vi "Get Data per Frequency at Pin Point Index.vi"(10 "Pin Point Index":i32, 11 "Full Data per Freq":string[][](array[string])) -> (3 "Focused Data":string[][](array[string]))   [LabVIEW 2023, in "FPT_Compression UI.lvlib"]
uses:
  FPT_Compression UI.lvlib
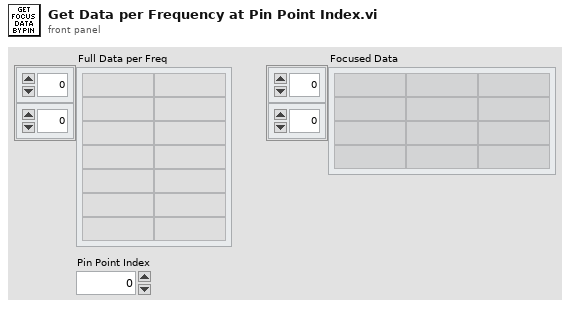
[diagram p1: front panel]
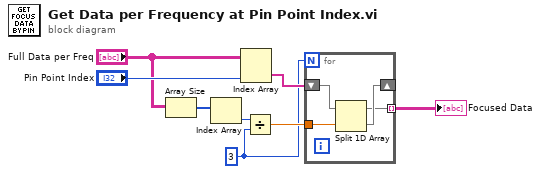
[diagram p0: block diagram]
diagram:
  w2 = 3 ("y")
  n1 = Array Size(array="Full Data per Freq") -> (size(s)=w3:i32[])
  n2 = Index Array(array=w3) -> (element=w6:i32)  [unwired: 1 in]
  n3 = Index Array(array="Full Data per Freq", index (col)="Pin Point Index") -> (element=w7:string[])  [unwired: 1 in]
  n4 = Divide(x=w6, y=w2) -> (x/y=w8:dbl)
  n5 = for {
    N: w2 -> [_]
    tunnel: [w11] -> w1 mode=indexing
    tunnel: w8 -> [w10]
    shift-right: [w12] -> _
    shift-left: w7 -> [w9]
    n6 = Split 1D Array(array=w9, index=w10) -> (first subarray=w11:string[], second subarray=w12:string[])
  }
  "Focused Data" <- w1
